vi "LoginSubVI.vi"(9 "Password":string, 10 "Username":string, 11 "file path (dialog if empty)":path) -> (3 "Status":bool)   [LabVIEW 2021]
uses:
  <vilib>/Utility/file.llb/Read Delimited Spreadsheet (string).vi
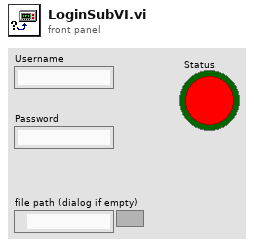
[diagram p1: front panel]
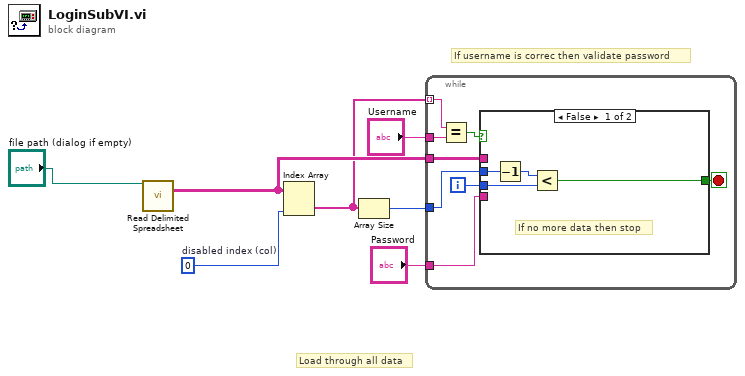
[diagram p0: block diagram]
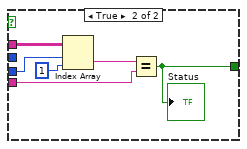
[diagram p2: hidden frame]
diagram:
  w1 = 0  # disabled index (col)
  # "If username is correc then validate password"
  # "Load through all data"
  n1 = call-poly <vilib>:"Read Delimited Spreadsheet.vi"("file path (dialog if empty)"="file path (dialog if empty)") -> ("all rows"=w4:string[][])  [unwired: 9 in, 5 out]
  n2 = Index Array "Index Array"(array=w4, index (col)=w1) -> (element=w2:string[])  [unwired: 1 in]
  n3 = Array Size(array=w2) -> (size(s)=w3:i32)
  n4 = while {
    tunnel: w2 -> [w11] mode=indexing
    tunnel: w4 -> [w15]
    tunnel: w3 -> [w13]
    tunnel: "Username" -> [w9]
    tunnel: "Password" -> [w8]
    i -> [w14]
    stop <- w12 stop-if-true
    n5 = Equal?(x=w11, y=w9) -> (x = y?=w10:bool)
    n6 = case shown="False" w10 {
      tunnel: w15 -> [_ w24]
      tunnel: w14 -> [w17 w23]
      tunnel: w13 -> [w19 _]
      tunnel: [w16 w25] -> w12
      tunnel: w8 -> [_ w20]
      frame False {
        # "If no more data then stop"
        n7 = Decrement(x=w19) -> (x-1=w18:i32)
        n8 = Less?(x=w18, y=w17) -> (x < y?=w16:bool)
      }
      frame True {
        n9 = Index Array "Index Array"(array=w24, index (row)=w23, index (col)=1 ("index")) -> (element=w21:string)
        n10 = Equal?(x=w21, y=w20) -> (x = y?=w25:bool)
        "Status" <- w25
      }
    }
  }
